vi "write_buffer_to_file.vi"(8 "error in (no error)":errorcluster, 10 "data_logger.lvclass":refnum<class "data_logger.lvclass">, 11 "detector in":refnum<class "detector.lvclass">) -> (0 "error out":errorcluster, 1 "Stream_done":bool, 2 "data_logger.lvclass 2":refnum<class "data_logger.lvclass">, 3 "detector out":refnum<class "detector.lvclass">)   [LabVIEW 2015, in "detector.lvclass"]
uses:
  detector.lvclass
  Data Logger Class/data_logger.lvclass
  detector.lvclass/detector.ctl
  lvoop_dll-master/picoquant_Tmodes.ctl
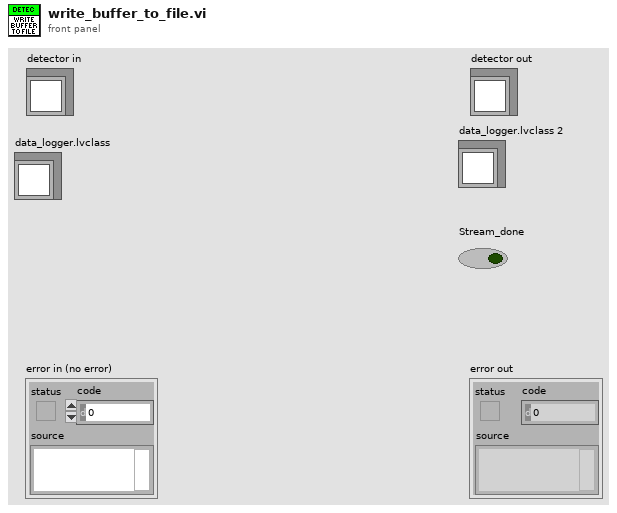
[diagram p1: front panel]
types:
  T1 = cluster{"stream":u64[], "channel":u8[], "sync":u64[], bool}
  T2 = typedef "picoquant_Tmodes.ctl" = u16
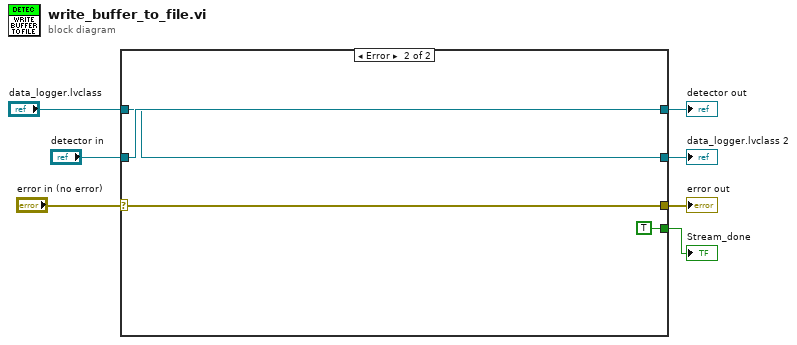
[diagram p0: block diagram]
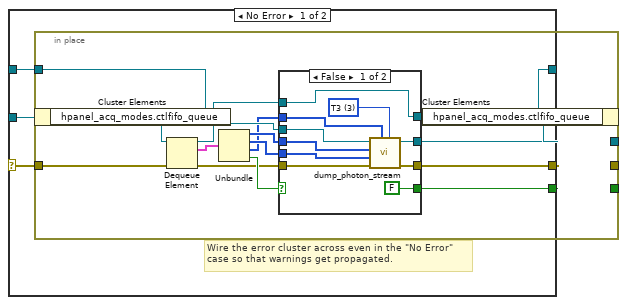
[diagram p2: hidden frame]
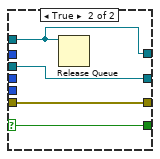
[diagram p3: hidden frame]
diagram:
  n1 = case shown="Error" "error in (no error)" {
    selector: "error in (no error)" -> [w11 w46]
    tunnel: [w9 w46] -> w6
    tunnel: [w8 w45] -> w4
    tunnel: "detector in" -> [w12 w45]
    tunnel: [w13 w44] -> w2
    tunnel: "data_logger.lvclass" -> [w14 w44]
    tunnel: [w10 TRUE] -> w1
    frame No Error {
      # "Wire the error cluster across even in the \"No Error\"\ncase so that warnings get propagated."
      n2 = in-place {
        in-place-border: w14 -> [w28]
        in-place-border: [w27] -> w13
        in-place-border: w11 -> [w25]
        in-place-border: [w22] -> w10
        in-place-border: [w17] -> w9
        n3 = in-place-cluster #1(w12) -> ("hpanel_acq_modes.ctlfifo_queue"=w26:refnum<queue>)
        n4 = Dequeue Element(queue=w26, error in (no error)=w25) -> (queue out=w16:refnum<queue>, element=w24:T1, error out=w18:errorcluster)  [unwired: 1 in, 1 out]
        n5 = Unbundle(w24) -> ("stream"=w21:u64[], "channel"=w20:u8[], "sync"=w19:u64[], w23:bool)
        n6 = case shown="False" w23 {
          selector: w23 -> [_ w42]
          tunnel: w28 -> [w38 w40]
          tunnel: [w37 w40] -> w27
          tunnel: [FALSE w42] -> w22
          tunnel: w21 -> [w35 _]
          tunnel: w20 -> [w34 _]
          tunnel: w19 -> [w33 _]
          tunnel: w18 -> [w31 w41]
          tunnel: [w30 w41] -> w17
          tunnel: w16 -> [w29 w39]
          tunnel: [w29 w39] -> w15
          frame False {
            w32 = T2 3 items=["T2"=2, "T3"=3] ("acq_mode")
            n7 = call-dynamic "dump_photon_stream.vi"("Ring"=w32, "sync"=w33, "error in (no error)"=w31, "channels"=w34, "photon_records"=w35, "data_logger in"=w38) -> ("error out"=w30:errorcluster, "data_logger out"=w37:refnum<class "data_logger.lvclass">)  [unwired: 4 in]
          }
          frame True {
            n8 = Release Queue(queue=w39) -> ()  [unwired: 2 in, 3 out]
          }
        }
        n9 = in-place-cluster #1("hpanel_acq_modes.ctlfifo_queue"=w15) -> (w8:refnum<class "detector.lvclass">)
      }
    }
    frame Error {
    }
  }
  "error out" <- w6
  "detector out" <- w4
  "data_logger.lvclass 2" <- w2
  "Stream_done" <- w1
